vi "getClassInfo.vi"(0 "reference in":refnum<class "DQMHModuleNode.lvclass">, 5 "error in (no error)":errorcluster) -> (9 "ClassPathUnmodified":path, 11 "methods(string)":string, 12 "Base class.bounds":T1 {"height" format="%.2f"; "width" format="%.2f"; "y" format="%.2f"; "x" format="%.2f"}, 13 "attributes(string)":string, 14 "reference out":refnum<class "DQMHModuleNode.lvclass">, 15 "className":string, 16 "attributes":string[](array[string]), 17 "methods":string[](array[string]), 18 "ClassPath":path, 19 "error out":errorcluster)   [LabVIEW 2014, in "DQMHModuleNode.lvclass"]
uses:
  <resource>/Framework/Providers/Open_GDS/UML/DQMHModuleNode_class/DQMHModuleNode.lvclass
  <resource>/Framework/Providers/Open_GDS/UML/General/Rectangle/Rectangle Rectangle2D.ctl
  <resource>/Framework/Providers/Open_GDS/UML/MultiLineString_class/MultiLineString.lvclass
  <resource>/Framework/Providers/Open_GDS/UML/RectangularNode_class/RectangularNode.lvclass
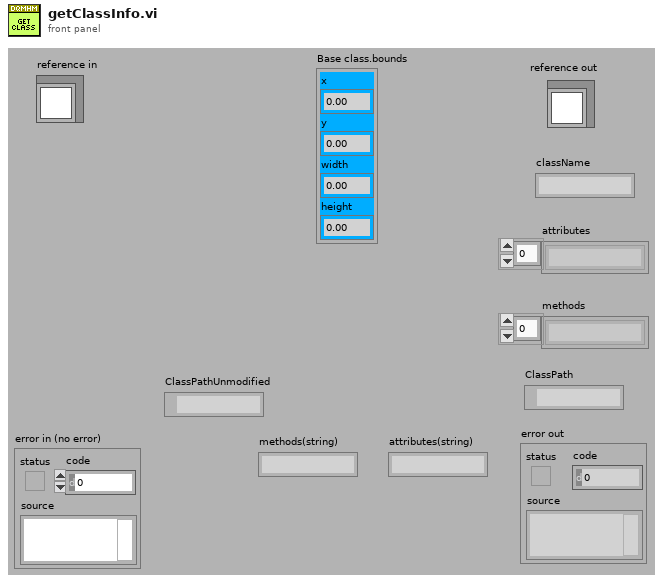
[diagram p1: front panel]
types:
  T1 = typedef "Rectangle Rectangle2D.ctl" = cluster{"x":dbl, "y":dbl, "width":dbl, "height":dbl}
  T2 = typedef "DQMHModuleNode.lvclass/ObjectAttributes.ctl" = cluster{"midHeight":dbl, "botHeight":dbl, "Name":refnum<class "MultiLineString.lvclass">, "Description":refnum<class "MultiLineString.lvclass">, "InternalData":refnum<class "MultiLineString.lvclass">, "Events":refnum<class "MultiLineString.lvclass">, "DEFAULT_COMPARTMENT_HEIGHT":i32, "DEFAULT_WIDTH":i32, "DEFAULT_HEIGHT":i32, "showEvents":bool, "showInternalData":bool, "ClassPath":path}
  T3 = typedef "RectangularNode.lvclass/ObjectAttributes.ctl" = cluster{"bounds":T1}
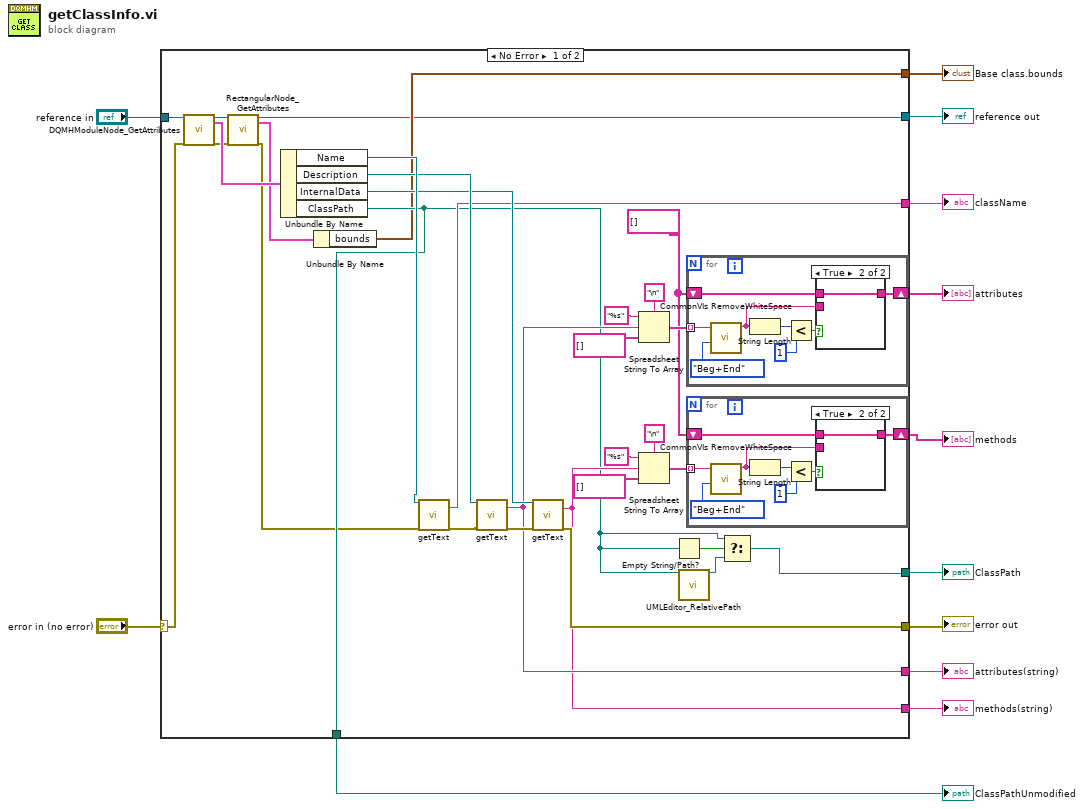
[diagram p0: block diagram]
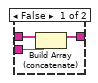
[diagram p2: hidden frame]
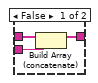
[diagram p3: hidden frame]
diagram:
  n1 = case shown="No Error" "error in (no error)" {
    selector: "error in (no error)" -> [w45 w70]
    tunnel: "reference in" -> [w44 w71]
    tunnel: [w41 w70] -> w10
    tunnel: [w14 w71] -> w9
    tunnel: [w37 _] -> w8
    tunnel: [w32 _] -> w7
    tunnel: [w27 _] -> w6
    tunnel: [w20 _] -> w5
    tunnel: [w25 _] -> w4
    tunnel: [w24 _] -> w3
    tunnel: [w22 _] -> w2
    tunnel: [w19 _] -> w1
    frame No Error {
      w26 = string[] []
      n2 = call <resource>:"DQMHModuleNode_GetAttributes.vi"("reference in"=w44, "error in (no error)"=w45) -> ("reference out"=w17:refnum<class "DQMHModuleNode.lvclass">, "Data"=w18:T2, "error out"=w16:errorcluster)  [unwired: 1 in, 14 out]
      n3 = call <resource>:"RectangularNode_GetAttributes.vi"("reference in"=w17, "error in (no error)"=w16) -> ("reference out"=w14:refnum<class "DQMHModuleNode.lvclass">, "Data"=w13:T3, "error out"=w15:errorcluster)  [unwired: 14 in, 1 out]
      n4 = Unbundle By Name(w18) -> ("Name"=w40:refnum<class "MultiLineString.lvclass">, "Description"=w39:refnum<class "MultiLineString.lvclass">, "InternalData"=w38:refnum<class "MultiLineString.lvclass">, "ClassPath"=w22:path)
      n5 = Unbundle By Name(w13) -> ("bounds"=w19:T1)
      n6 = call-dynamic "getText.vi"("reference"=w40, "error in (no error)"=w15) -> ("text"=w37:string, "error out"=w43:errorcluster)  [unwired: 16 out]
      n7 = call-dynamic "getText.vi"("reference"=w39, "error in (no error)"=w43) -> ("text"=w25:string, "error out"=w42:errorcluster)  [unwired: 16 out]
      n8 = call-dynamic "getText.vi"("reference"=w38, "error in (no error)"=w42) -> ("text"=w24:string, "error out"=w41:errorcluster)  [unwired: 16 out]
      n9 = Spreadsheet String To Array(delimiter (Tab)="\n", format string="%s", spreadsheet string=w25, array type (2D Dbl)=string[] []) -> (array=w33:string[])
      n10 = Spreadsheet String To Array(delimiter (Tab)="\n", format string="%s", spreadsheet string=w24, array type (2D Dbl)=string[] []) -> (array=w31:string[])
      n11 = Empty String/Path?(string/path=w22) -> (empty?=w23:bool)
      n12 = call <resource>:"UMLEditor_RelativePath.vi"("Path In"=w22) -> ("ConvertToAbsolutePath(If possible)"=w21:path)  [unwired: 1 in, 17 out]
      n13 = for {
        tunnel: w33 -> [w65] mode=indexing
        shift-right: [w58] -> w32
        shift-left: w26 -> [w60]
        n14 = call <resource>:"CommonVIs RemoveWhiteSpace.vi"("Remove from"=enum16{"Begining", "End", "Beg+End", "All"}."Beg+End", "String in"=w65) -> ("String out"=w59:string)  [unwired: 2 in, 3 out]
        n15 = String Length(string=w59) -> (length=w63:i32)
        n16 = Less?(x=w63, y=1) -> (x < y?=w61:bool)
        n17 = case shown="True" w61 {
          tunnel: w60 -> [w68 w69]
          tunnel: w59 -> [w67 _]
          tunnel: [w66 w69] -> w58
          frame False {
            n18 = Build Array (concatenate)(w68, w67) -> (w66:string[])
          }
          frame True {
          }
        }
      }
      n19 = for {
        tunnel: w31 -> [w53] mode=indexing
        shift-right: [w46] -> w27
        shift-left: w26 -> [w48]
        n20 = call <resource>:"CommonVIs RemoveWhiteSpace.vi"("Remove from"=enum16{"Begining", "End", "Beg+End", "All"}."Beg+End", "String in"=w53) -> ("String out"=w47:string)  [unwired: 2 in, 3 out]
        n21 = String Length(string=w47) -> (length=w51:i32)
        n22 = Less?(x=w51, y=1) -> (x < y?=w49:bool)
        n23 = case shown="True" w49 {
          tunnel: w48 -> [w56 w57]
          tunnel: w47 -> [w55 _]
          tunnel: [w54 w57] -> w46
          frame False {
            n24 = Build Array (concatenate)(w56, w55) -> (w54:string[])
          }
          frame True {
          }
        }
      }
      n25 = Select(t=w22, s=w23, f=w21) -> (s? t:f=w20:path)
    }
    frame Error {
    }
  }
  "reference out" <- w9
  "error out" <- w10
  "className" <- w8
  "attributes" <- w7
  "methods" <- w6
  "ClassPath" <- w5
  "attributes(string)" <- w4
  "methods(string)" <- w3
  "ClassPathUnmodified" <- w2
  "Base class.bounds" <- w1
